vi "Communicator - Passive2.v.vi"() -> ()   [LabVIEW 2019]
panel:
  out "BL_Receive":T1 {"ControlScheme"."Time" format="%<%Y-%m-%d %H:%M:%S>T"; "ControllerConfig"."Time" format="%<%Y-%m-%d %H:%M:%S>T"; "BalancingMotor-All"."BalancingMotor-00"."Time" format="%<%Y-%m-%d %H:%M:%S>T"; "BalancingMotor-All"."BalancingMotor-01"."Time" format="%<%Y-%m-%d %H:%M:%S>T"; "BalancingMotor-All"."BalancingMotor-02"."Time" format="%<%Y-%m-%d %H:%M:%S>T"; "BalancingMotor-All"."BalancingMotor-03"."Time" format="%<%Y-%m-%d %H:%M:%S>T"}
  in  "BL_Send":T1 {"ControlScheme"."Time" format="%<%Y-%m-%d %H:%M:%S>T"; "ControllerConfig"."Time" format="%<%Y-%m-%d %H:%M:%S>T"; "BalancingMotor-All"."BalancingMotor-00"."Time" format="%<%Y-%m-%d %H:%M:%S>T"; "BalancingMotor-All"."BalancingMotor-01"."Time" format="%<%Y-%m-%d %H:%M:%S>T"; "BalancingMotor-All"."BalancingMotor-02"."Time" format="%<%Y-%m-%d %H:%M:%S>T"; "BalancingMotor-All"."BalancingMotor-03"."Time" format="%<%Y-%m-%d %H:%M:%S>T"}
  out "BL_Send2":T1 {"ControlScheme"."Time" format="%<%Y-%m-%d %H:%M:%S>T"; "ControllerConfig"."Time" format="%<%Y-%m-%d %H:%M:%S>T"; "BalancingMotor-All"."BalancingMotor-00"."Time" format="%<%Y-%m-%d %H:%M:%S>T"; "BalancingMotor-All"."BalancingMotor-01"."Time" format="%<%Y-%m-%d %H:%M:%S>T"; "BalancingMotor-All"."BalancingMotor-02"."Time" format="%<%Y-%m-%d %H:%M:%S>T"; "BalancingMotor-All"."BalancingMotor-03"."Time" format="%<%Y-%m-%d %H:%M:%S>T"}
  in  "Port":u16=6343
  in  "stop":bool
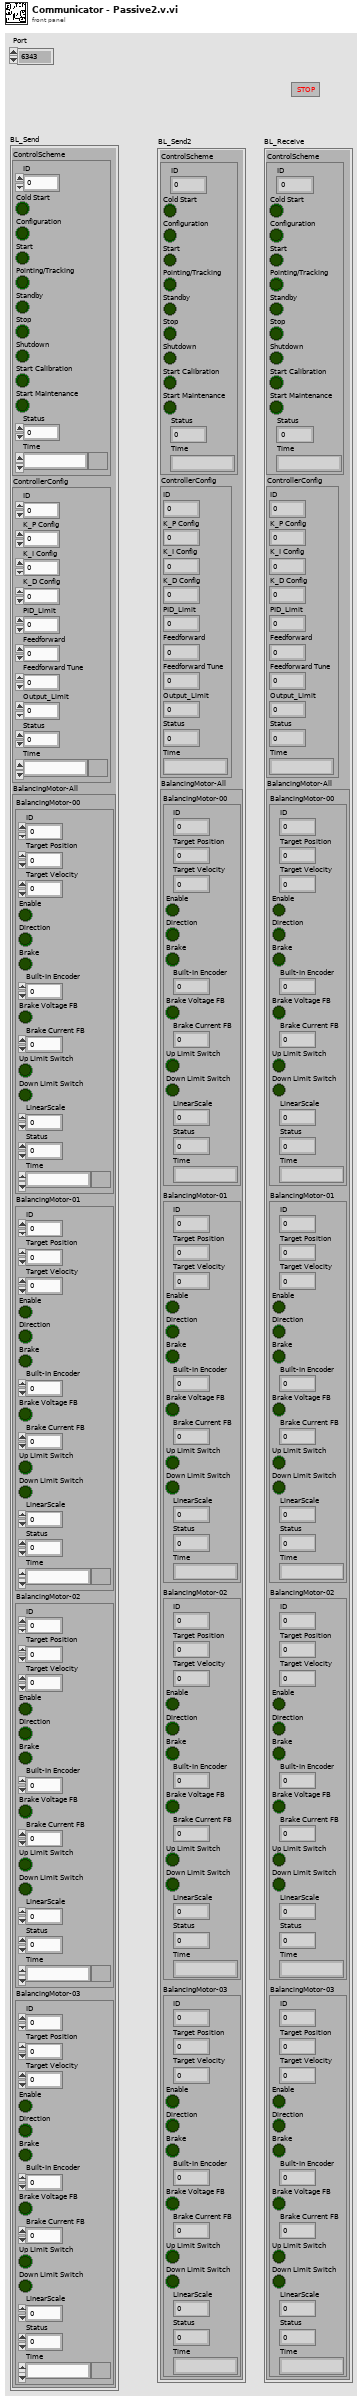
[diagram p1: front panel]
types:
  T1 = cluster{"ControlScheme":cluster{"ID":i32, "Cold Start":bool, "Configuration":bool, "Start":bool, "Pointing/Tracking":bool, "Standby":bool, "Stop":bool, "Shutdown":bool, "Start Calibration":bool, "Start Maintenance":bool, "Status":i16, "Time ":timestamp}, "ControllerConfig":cluster{"ID":i32, "K_P Config":u64, "K_I Config":u64, "K_D Config":u64, "PID_Limit":u64, "Feedforward":u64, "Feedforward Tune":u64, "Output_Limit":u64, "Status":i16, "Time ":timestamp}, "BalancingMotor-All":cluster{"BalancingMotor-00":cluster{"ID":i32, "Target Position":u64, "Target Velocity":u64, "Enable":bool, "Direction":bool, "Brake":bool, "Built-In Encoder":u64, "Brake Voltage FB":bool, "Brake Current FB":u64, "Up Limit Switch":bool, "Down Limit Switch":bool, "LinearScale":u64, "Status":i16, "Time ":timestamp}, "BalancingMotor-01":cluster{"ID":i32, "Target Position":u64, "Target Velocity":u64, "Enable":bool, "Direction":bool, "Brake":bool, "Built-In Encoder":u64, "Brake Voltage FB":bool, "Brake Current FB":u64, "Up Limit Switch":bool, "Down Limit Switch":bool, "LinearScale":u64, "Status":i16, "Time ":timestamp}, "BalancingMotor-02":cluster{"ID":i32, "Target Position":u64, "Target Velocity":u64, "Enable":bool, "Direction":bool, "Brake":bool, "Built-In Encoder":u64, "Brake Voltage FB":bool, "Brake Current FB":u64, "Up Limit Switch":bool, "Down Limit Switch":bool, "LinearScale":u64, "Status":i16, "Time ":timestamp}, "BalancingMotor-03":cluster{"ID":i32, "Target Position":u64, "Target Velocity":u64, "Enable":bool, "Direction":bool, "Brake":bool, "Built-In Encoder":u64, "Brake Voltage FB":bool, "Brake Current FB":u64, "Up Limit Switch":bool, "Down Limit Switch":bool, "LinearScale":u64, "Status":i16, "Time ":timestamp}}}
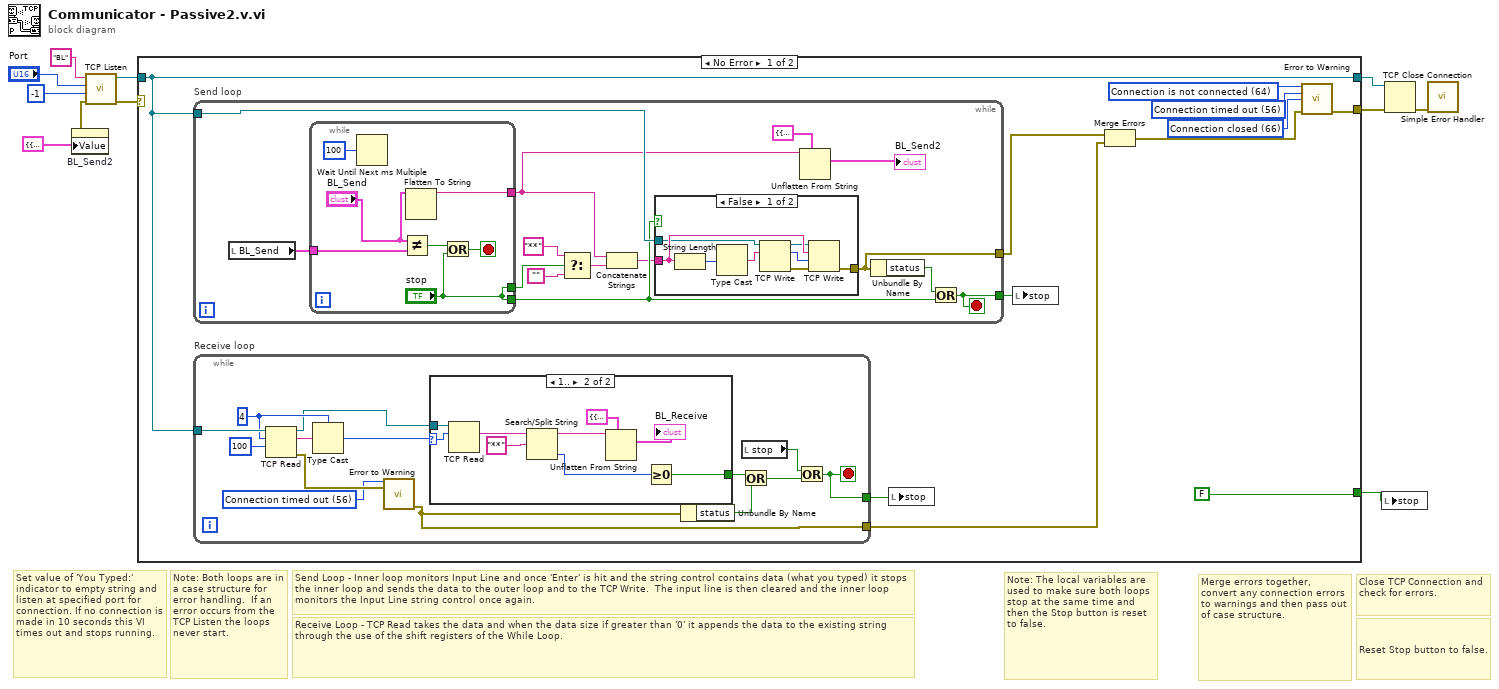
[diagram p0: block diagram]
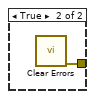
[diagram p2: hidden frame]
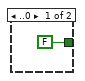
[diagram p3: hidden frame]
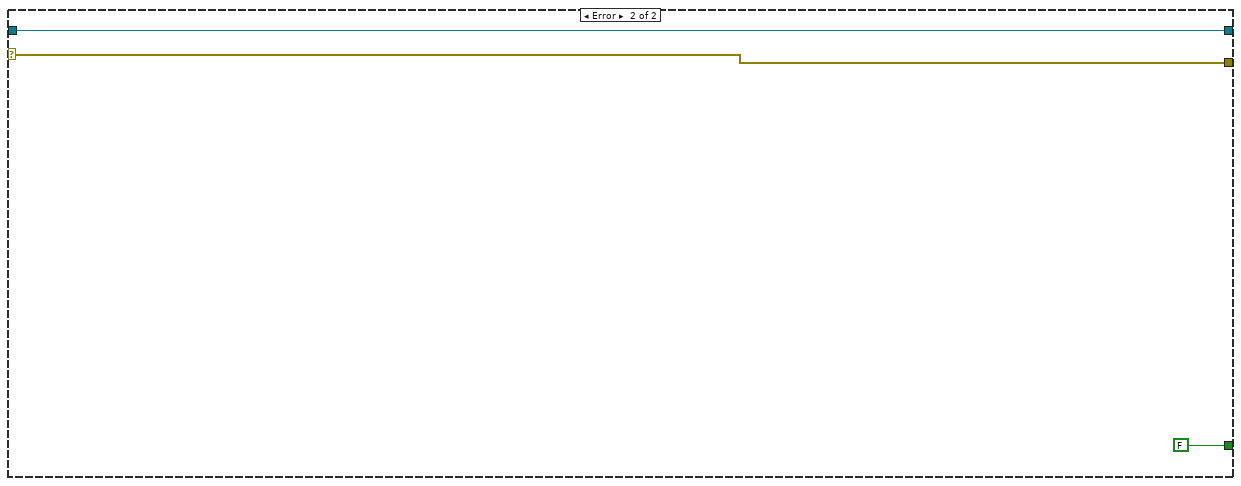
[diagram p4: hidden frame]
diagram:
  # "Reset Stop button to false."
  # "Close TCP Connection and check for errors."
  # "Note: Both loops are in a case structure for error handling.  If an error occurs from the TCP Listen the loops never start."
  # "Merge errors together, convert any connection errors to warnings and then pass out of case structure."
  # "Note: The local variables are used to make sure both loops stop at the same time and then the Stop button is reset to false."
  # "Receive Loop - TCP Read takes the data and when the data size if greater than '0' it appends the data to the existing string through the use of the shift registers of the While Loop."
  # "Send Loop - Inner loop monitors Input Line and once 'Enter' is hit and the string control contains data (what you typed) it stops the inner loop and sends the data to the outer loop and to the TCP Write.  The input line is then cleared and the inner loop monitors the Input Line string control once again."
  # "Set value of 'You Typed:' indicator to empty string and listen at specified port for connection. If no connection is made in 10 seconds this VI times out and stops running."
  n1 = property on="BL_Send2" class="Clust (strict)"("Value"=T1 {"ControlScheme"={"ID"=0, "Cold Start"=FALSE, "Configuration"=FALSE, "Start"=FALSE, "Pointing/Tracking"=FALSE, "Standby"=FALSE, "Stop"=FALSE, "Shutdown"=FALSE, "Start Calibration"=FALSE, "Start Maintenance"=FALSE, "Status"=0, "Time "=timestamp(0 s since 1904-01-01)}, "ControllerConfig"={"ID"=0, "K_P Config"=0, "K_I Config"=0, "K_D Config"=0, "PID_Limit"=0, "Feedforward"=0, "Feedforward Tune"=0, "Output_Limit"=0, "Status"=0, "Time "=timestamp(0 s since 1904-01-01)}, "BalancingMotor-All"={"BalancingMotor-00"={"ID"=0, "Target Position"=0, "Target Velocity"=0, "Enable"=FALSE, "Direction"=FALSE, "Brake"=FALSE, "Built-In Encoder"=0, "Brake Voltage FB"=FALSE, "Brake Current FB"=0, "Up Limit Switch"=FALSE, "Down Limit Switch"=FALSE, "LinearScale"=0, "Status"=0, "Time "=timestamp(0 s since 1904-01-01)}, "BalancingMotor-01"={"ID"=0, "Target Position"=0, "Target Velocity"=0, "Enable"=FALSE, "Direction"=FALSE, "Brake"=FALSE, "Built-In Encoder"=0, "Brake Voltage FB"=FALSE, "Brake Current FB"=0, "Up Limit Switch"=FALSE, "Down Limit Switch"=FALSE, "LinearScale"=0, "Status"=0, "Time "=timestamp(0 s since 1904-01-01)}, "BalancingMotor-02"={"ID"=0, "Target Position"=0, "Target Velocity"=0, "Enable"=FALSE, "Direction"=FALSE, "Brake"=FALSE, "Built-In Encoder"=0, "Brake Voltage FB"=FALSE, "Brake Current FB"=0, "Up Limit Switch"=FALSE, "Down Limit Switch"=FALSE, "LinearScale"=0, "Status"=0, "Time "=timestamp(0 s since 1904-01-01)}, "BalancingMotor-03"={"ID"=0, "Target Position"=0, "Target Velocity"=0, "Enable"=FALSE, "Direction"=FALSE, "Brake"=FALSE, "Built-In Encoder"=0, "Brake Voltage FB"=FALSE, "Brake Current FB"=0, "Up Limit Switch"=FALSE, "Down Limit Switch"=FALSE, "LinearScale"=0, "Status"=0, "Time "=timestamp(0 s since 1904-01-01)}}} ("BL_Send")) -> (error out=w1:errorcluster)  [unwired: 2 in, 1 out]
  n2 = call <vilib>:"TCP Listen.vi"("error in (no error)"=w1, "timeout ms (wait forever: -1)"=-1, "port"="Port", "service name"="BL") -> ("error out"=w7:errorcluster, "connection ID"=w8:refnum<k5>)  [unwired: 3 in, 3 out]
  n3 = case shown="No Error" w7 {
    selector: w7 -> [_ w78]
    tunnel: [w17 w78] -> w10
    tunnel: w8 -> [w12 w79]
    tunnel: [w12 w79] -> w11
    tunnel: [FALSE FALSE] -> w4
    frame No Error {
      w14 = 56 items=["No Error", "Argument Error", "Memory Full", "Out of Zone", "End of File", "File Already Open", "Generic File IO Error", "File Not Found", "File Permission Error", "Disk Full", "Duplicate Path", "Too Many Files Open", "Not Enabled", "Resource File Not Found", "Cannot Add Resource", "Resource Not Found", "Image Not Found", "Image Memory Error", "Pen Does Not Exist", "Config Bad Type", "Config Token Not Found", "Config Parse Error", "Config Memory Error", "Bad External Code Format", "Bad External Code Offset", "External Code Not Present", "Null Window", "Destroy Window Mixup", "Null Menu", "Print Aborted", "Bad Print Record", "Print Driver Error", "Windows Error During Print", "Memory Error During Print", "Print Dialog Error", "Generic Print Error", "Invalid Device Refnum", "Device Not Found", "Device Parameter Error", "Device Unit Error", "Can't Open Device", "Device Call Aborted", "Generic Error", "Cancelled By User", "Object ID Too Low", "Object ID Too High", "Object Not In Heap", "Unknown Heap", "Bad DefProc ID", "DefProc Not In Table", "Message Out Of Range", "Null Method", "Unknown Message", "Manager Call Not Supported", "Bad address", "Connection In progress", "Connection timed out", "Connection is already in progress", "Network attribute not supported", "Network error", "Address in use", "System out of memory", "Connection aborted", "Connection refused", "Connection is not connected", "Connection is already connected", "Connection closed", "Initialize error (interapplication manager)", "Bad occurrence", "Wait on unbound occurrence handler", "Occurrence queue overflow", "Bad path", "Semaphore not signaled", "Unrecognized type (interapplication manager)"] ("2nd Error to Convert")
      w18 = 66 items=["No Error", "Argument Error", "Memory Full", "Out of Zone", "End of File", "File Already Open", "Generic File IO Error", "File Not Found", "File Permission Error", "Disk Full", "Duplicate Path", "Too Many Files Open", "Not Enabled", "Resource File Not Found", "Cannot Add Resource", "Resource Not Found", "Image Not Found", "Image Memory Error", "Pen Does Not Exist", "Config Bad Type", "Config Token Not Found", "Config Parse Error", "Config Memory Error", "Bad External Code Format", "Bad External Code Offset", "External Code Not Present", "Null Window", "Destroy Window Mixup", "Null Menu", "Print Aborted", "Bad Print Record", "Print Driver Error", "Windows Error During Print", "Memory Error During Print", "Print Dialog Error", "Generic Print Error", "Invalid Device Refnum", "Device Not Found", "Device Parameter Error", "Device Unit Error", "Can't Open Device", "Device Call Aborted", "Generic Error", "Cancelled By User", "Object ID Too Low", "Object ID Too High", "Object Not In Heap", "Unknown Heap", "Bad DefProc ID", "DefProc Not In Table", "Message Out Of Range", "Null Method", "Unknown Message", "Manager Call Not Supported", "Bad address", "Connection In progress", "Connection timed out", "Connection is already in progress", "Network attribute not supported", "Network error", "Address in use", "System out of memory", "Connection aborted", "Connection refused", "Connection is not connected", "Connection is already connected", "Connection closed", "Initialize error (interapplication manager)", "Bad occurrence", "Wait on unbound occurrence handler", "Occurrence queue overflow", "Bad path", "Semaphore not signaled", "Unrecognized type (interapplication manager)"] ("3rd Error to Convert")
      w19 = 64 items=["No Error", "Argument Error", "Memory Full", "Out of Zone", "End of File", "File Already Open", "Generic File IO Error", "File Not Found", "File Permission Error", "Disk Full", "Duplicate Path", "Too Many Files Open", "Not Enabled", "Resource File Not Found", "Cannot Add Resource", "Resource Not Found", "Image Not Found", "Image Memory Error", "Pen Does Not Exist", "Config Bad Type", "Config Token Not Found", "Config Parse Error", "Config Memory Error", "Bad External Code Format", "Bad External Code Offset", "External Code Not Present", "Null Window", "Destroy Window Mixup", "Null Menu", "Print Aborted", "Bad Print Record", "Print Driver Error", "Windows Error During Print", "Memory Error During Print", "Print Dialog Error", "Generic Print Error", "Invalid Device Refnum", "Device Not Found", "Device Parameter Error", "Device Unit Error", "Can't Open Device", "Device Call Aborted", "Generic Error", "Cancelled By User", "Object ID Too Low", "Object ID Too High", "Object Not In Heap", "Unknown Heap", "Bad DefProc ID", "DefProc Not In Table", "Message Out Of Range", "Null Method", "Unknown Message", "Manager Call Not Supported", "Bad address", "Connection In progress", "Connection timed out", "Connection is already in progress", "Network attribute not supported", "Network error", "Address in use", "System out of memory", "Connection aborted", "Connection refused", "Connection is not connected", "Connection is already connected", "Connection closed", "Initialize error (interapplication manager)", "Bad occurrence", "Wait on unbound occurrence handler", "Occurrence queue overflow", "Bad path", "Semaphore not signaled", "Unrecognized type (interapplication manager)"] ("1st Error to Convert")
      n4 = while "Send loop" {
        tunnel: w12 -> [w35]
        tunnel: [w36] -> w15
        tunnel: [w31] -> w21
        stop <- w36 stop-if-true
        n5 = local read "BL_Send"() -> (w28:T1)
        n6 = while {
          tunnel: ["stop"] -> w33
          tunnel: ["stop"] -> w29
          tunnel: [w38] -> w27
          tunnel: w28 -> [w40]
          stop <- w41 stop-if-true
          n7 = Wait Until Next ms Multiple(millisecond multiple=u32 100) -> ()  [unwired: 1 out]
          n8 = Not Equal?(x="BL_Send", y=w40) -> (x != y?=w42:bool)
          n9 = Flatten To String(anything="BL_Send") -> (data string=w38:string)  [unwired: 3 in, 2 out]
          n10 = Or(x=w42, y="stop") -> (x .or. y?=w41:bool)
        }
        n11 = Select(t="**", s=w33, f="") -> (s? t:f=w26:string)
        n12 = Concatenate Strings(w27, w26) -> (w25:string)
        n13 = case shown="False" w29 {
          tunnel: w25 -> [w48 _]
          tunnel: [w51 w52] -> w31
          tunnel: w35 -> [w45 _]
          frame False {
            n14 = String Length(string=w48) -> (length=w47:i32)
            n15 = Type Cast(x=w47) -> (*(type *) &x=w46:string)  [unwired: 1 in]
            n16 = TCP Write(connection ID=w45, data in=w46) -> (connection ID out=w44:refnum<k5>, bytes written=w49:i32, error out=w50:errorcluster)  [unwired: 2 in]
            n17 = TCP Write(connection ID=w44, data in=w48, error in (no error)=w50, 9:w49) -> (error out=w51:errorcluster)  [unwired: 2 out]
          }
          frame True {
            n18 = call <vilib>:"Clear Errors.vi"() -> ("error out"=w52:errorcluster)  [unwired: 6 in, 1 out]
          }
        }
        n19 = Unflatten From String(type=T1 {"ControlScheme"={"ID"=0, "Cold Start"=FALSE, "Configuration"=FALSE, "Start"=FALSE, "Pointing/Tracking"=FALSE, "Standby"=FALSE, "Stop"=FALSE, "Shutdown"=FALSE, "Start Calibration"=FALSE, "Start Maintenance"=FALSE, "Status"=0, "Time "=timestamp(0 s since 1904-01-01)}, "ControllerConfig"={"ID"=0, "K_P Config"=0, "K_I Config"=0, "K_D Config"=0, "PID_Limit"=0, "Feedforward"=0, "Feedforward Tune"=0, "Output_Limit"=0, "Status"=0, "Time "=timestamp(0 s since 1904-01-01)}, "BalancingMotor-All"={"BalancingMotor-00"={"ID"=0, "Target Position"=0, "Target Velocity"=0, "Enable"=FALSE, "Direction"=FALSE, "Brake"=FALSE, "Built-In Encoder"=0, "Brake Voltage FB"=FALSE, "Brake Current FB"=0, "Up Limit Switch"=FALSE, "Down Limit Switch"=FALSE, "LinearScale"=0, "Status"=0, "Time "=timestamp(0 s since 1904-01-01)}, "BalancingMotor-01"={"ID"=0, "Target Position"=0, "Target Velocity"=0, "Enable"=FALSE, "Direction"=FALSE, "Brake"=FALSE, "Built-In Encoder"=0, "Brake Voltage FB"=FALSE, "Brake Current FB"=0, "Up Limit Switch"=FALSE, "Down Limit Switch"=FALSE, "LinearScale"=0, "Status"=0, "Time "=timestamp(0 s since 1904-01-01)}, "BalancingMotor-02"={"ID"=0, "Target Position"=0, "Target Velocity"=0, "Enable"=FALSE, "Direction"=FALSE, "Brake"=FALSE, "Built-In Encoder"=0, "Brake Voltage FB"=FALSE, "Brake Current FB"=0, "Up Limit Switch"=FALSE, "Down Limit Switch"=FALSE, "LinearScale"=0, "Status"=0, "Time "=timestamp(0 s since 1904-01-01)}, "BalancingMotor-03"={"ID"=0, "Target Position"=0, "Target Velocity"=0, "Enable"=FALSE, "Direction"=FALSE, "Brake"=FALSE, "Built-In Encoder"=0, "Brake Voltage FB"=FALSE, "Brake Current FB"=0, "Up Limit Switch"=FALSE, "Down Limit Switch"=FALSE, "LinearScale"=0, "Status"=0, "Time "=timestamp(0 s since 1904-01-01)}}} ("BL_Send"), binary string=w27) -> (value=→"BL_Send2":T1)  [unwired: 3 in, 2 out]
        n20 = Unbundle By Name(w31) -> ("status"=w30:bool)
        n21 = Or(x=w30, y=w29) -> (x .or. y?=w36:bool)
      }
      n22 = while "Receive loop" {
        tunnel: [w65] -> w16
        tunnel: [w60] -> w22
        tunnel: w12 -> [w66]
        stop <- w65 stop-if-true
        w55 = 4
        w61 = 56 items=["No Error", "Argument Error", "Memory Full", "Out of Zone", "End of File", "File Already Open", "Generic File IO Error", "File Not Found", "File Permission Error", "Disk Full", "Duplicate Path", "Too Many Files Open", "Not Enabled", "Resource File Not Found", "Cannot Add Resource", "Resource Not Found", "Image Not Found", "Image Memory Error", "Pen Does Not Exist", "Config Bad Type", "Config Token Not Found", "Config Parse Error", "Config Memory Error", "Bad External Code Format", "Bad External Code Offset", "External Code Not Present", "Null Window", "Destroy Window Mixup", "Null Menu", "Print Aborted", "Bad Print Record", "Print Driver Error", "Windows Error During Print", "Memory Error During Print", "Print Dialog Error", "Generic Print Error", "Invalid Device Refnum", "Device Not Found", "Device Parameter Error", "Device Unit Error", "Can't Open Device", "Device Call Aborted", "Generic Error", "Cancelled By User", "Object ID Too Low", "Object ID Too High", "Object Not In Heap", "Unknown Heap", "Bad DefProc ID", "DefProc Not In Table", "Message Out Of Range", "Null Method", "Unknown Message", "Manager Call Not Supported", "Bad address", "Connection In progress", "Connection timed out", "Connection is already in progress", "Network attribute not supported", "Network error", "Address in use", "System out of memory", "Connection aborted", "Connection refused", "Connection is not connected", "Connection is already connected", "Connection closed", "Initialize error (interapplication manager)", "Bad occurrence", "Wait on unbound occurrence handler", "Occurrence queue overflow", "Bad path", "Semaphore not signaled", "Unrecognized type (interapplication manager)"] ("1st Error to Convert")
        n23 = TCP Read(connection ID=w66, bytes to read=w55, 9:100) -> (connection ID out=w53:refnum<k5>, data out=w56:string, error out=w62:errorcluster)  [unwired: 2 in]
        n24 = Type Cast(type=w55, x=w56) -> (*(type *) &x=w54:i32)
        n25 = call <vilib>:"Error to Warning.vi"("1st Error to Convert"=w61, "error in"=w62) -> ("warning out"=w60:errorcluster)  [unwired: 13 in]
        n26 = case shown="1.." w54 {
          selector: w54 -> [_ w76]
          tunnel: [FALSE w72] -> w64
          tunnel: w53 -> [_ w75]
          frame ..0 {
          }
          frame 1.. {
            n27 = TCP Read(connection ID=w75, bytes to read=w76) -> (data out=w69:string)  [unwired: 3 in, 2 out]
            n28 = Search/Split String(string=w69, search string/char (-)="**") -> (substring before match=w68:string, offset of match=w74:i32)  [unwired: 1 in, 1 out]
            n29 = Unflatten From String(type=T1 {"ControlScheme"={"ID"=0, "Cold Start"=FALSE, "Configuration"=FALSE, "Start"=FALSE, "Pointing/Tracking"=FALSE, "Standby"=FALSE, "Stop"=FALSE, "Shutdown"=FALSE, "Start Calibration"=FALSE, "Start Maintenance"=FALSE, "Status"=0, "Time "=timestamp(0 s since 1904-01-01)}, "ControllerConfig"={"ID"=0, "K_P Config"=0, "K_I Config"=0, "K_D Config"=0, "PID_Limit"=0, "Feedforward"=0, "Feedforward Tune"=0, "Output_Limit"=0, "Status"=0, "Time "=timestamp(0 s since 1904-01-01)}, "BalancingMotor-All"={"BalancingMotor-00"={"ID"=0, "Target Position"=0, "Target Velocity"=0, "Enable"=FALSE, "Direction"=FALSE, "Brake"=FALSE, "Built-In Encoder"=0, "Brake Voltage FB"=FALSE, "Brake Current FB"=0, "Up Limit Switch"=FALSE, "Down Limit Switch"=FALSE, "LinearScale"=0, "Status"=0, "Time "=timestamp(0 s since 1904-01-01)}, "BalancingMotor-01"={"ID"=0, "Target Position"=0, "Target Velocity"=0, "Enable"=FALSE, "Direction"=FALSE, "Brake"=FALSE, "Built-In Encoder"=0, "Brake Voltage FB"=FALSE, "Brake Current FB"=0, "Up Limit Switch"=FALSE, "Down Limit Switch"=FALSE, "LinearScale"=0, "Status"=0, "Time "=timestamp(0 s since 1904-01-01)}, "BalancingMotor-02"={"ID"=0, "Target Position"=0, "Target Velocity"=0, "Enable"=FALSE, "Direction"=FALSE, "Brake"=FALSE, "Built-In Encoder"=0, "Brake Voltage FB"=FALSE, "Brake Current FB"=0, "Up Limit Switch"=FALSE, "Down Limit Switch"=FALSE, "LinearScale"=0, "Status"=0, "Time "=timestamp(0 s since 1904-01-01)}, "BalancingMotor-03"={"ID"=0, "Target Position"=0, "Target Velocity"=0, "Enable"=FALSE, "Direction"=FALSE, "Brake"=FALSE, "Built-In Encoder"=0, "Brake Voltage FB"=FALSE, "Brake Current FB"=0, "Up Limit Switch"=FALSE, "Down Limit Switch"=FALSE, "LinearScale"=0, "Status"=0, "Time "=timestamp(0 s since 1904-01-01)}}} ("BL_Send"), binary string=w68) -> (value=→"BL_Receive":T1)  [unwired: 3 in, 2 out]
            n30 = Greater Or Equal To 0?(x=w74) -> (x >= 0?=w72:bool)
          }
        }
        n31 = Unbundle By Name(w60) -> ("status"=w59:bool)
        n32 = Or(x=w64, y=w59) -> (x .or. y?=w57:bool)
        n33 = local read "stop"() -> (w58:bool)
        n34 = Or(x=w58, y=w57) -> (x .or. y?=w65:bool)
      }
      n35 = local write "stop"(w16) -> ()
      n36 = local write "stop"(w15) -> ()
      n37 = Merge Errors(w21, w22) -> (w20:errorcluster)
      n38 = call <vilib>:"Error to Warning.vi"("1st Error to Convert"=w19, "2nd Error to Convert"=w14, "3rd Error to Convert"=w18, "error in"=w20) -> ("warning out"=w17:errorcluster)  [unwired: 11 in]
    }
    frame Error {
    }
  }
  n39 = local write "stop"(w4) -> ()
  n40 = TCP Close Connection(connection ID=w11, error in (no error)=w10) -> (error out=w9:errorcluster)  [unwired: 1 in, 1 out]
  n41 = call <vilib>:"Simple Error Handler.vi"("error in (no error)"=w9) -> ()  [unwired: 4 in, 5 out]
